vi "MesswertePlotten.vi"(0 "Intensity 0-100":dbl(knob) min=0.0 max=100.0 step=1.0 scale=0.0..100.0, 1 "VISA resource name":refnum<visa-resource-name>, 2 "file path (use dialog)":path, 3 "Upper colourlimit Temperatur":u32(colorbox), 4 "Lower colourlimit Temperatur":u32(colorbox), 5 "Upper colourlimit Humidity":u32(colorbox), 6 "Lower colourlimit Humidity":u32(colorbox)) -> ()   [LabVIEW 2021]
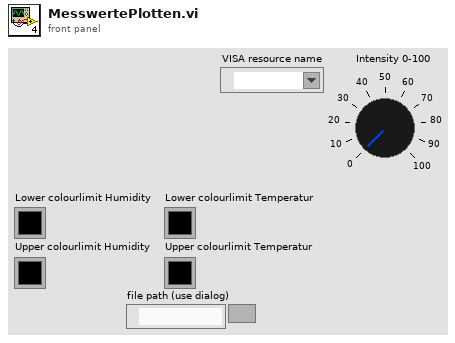
[diagram p1: front panel]
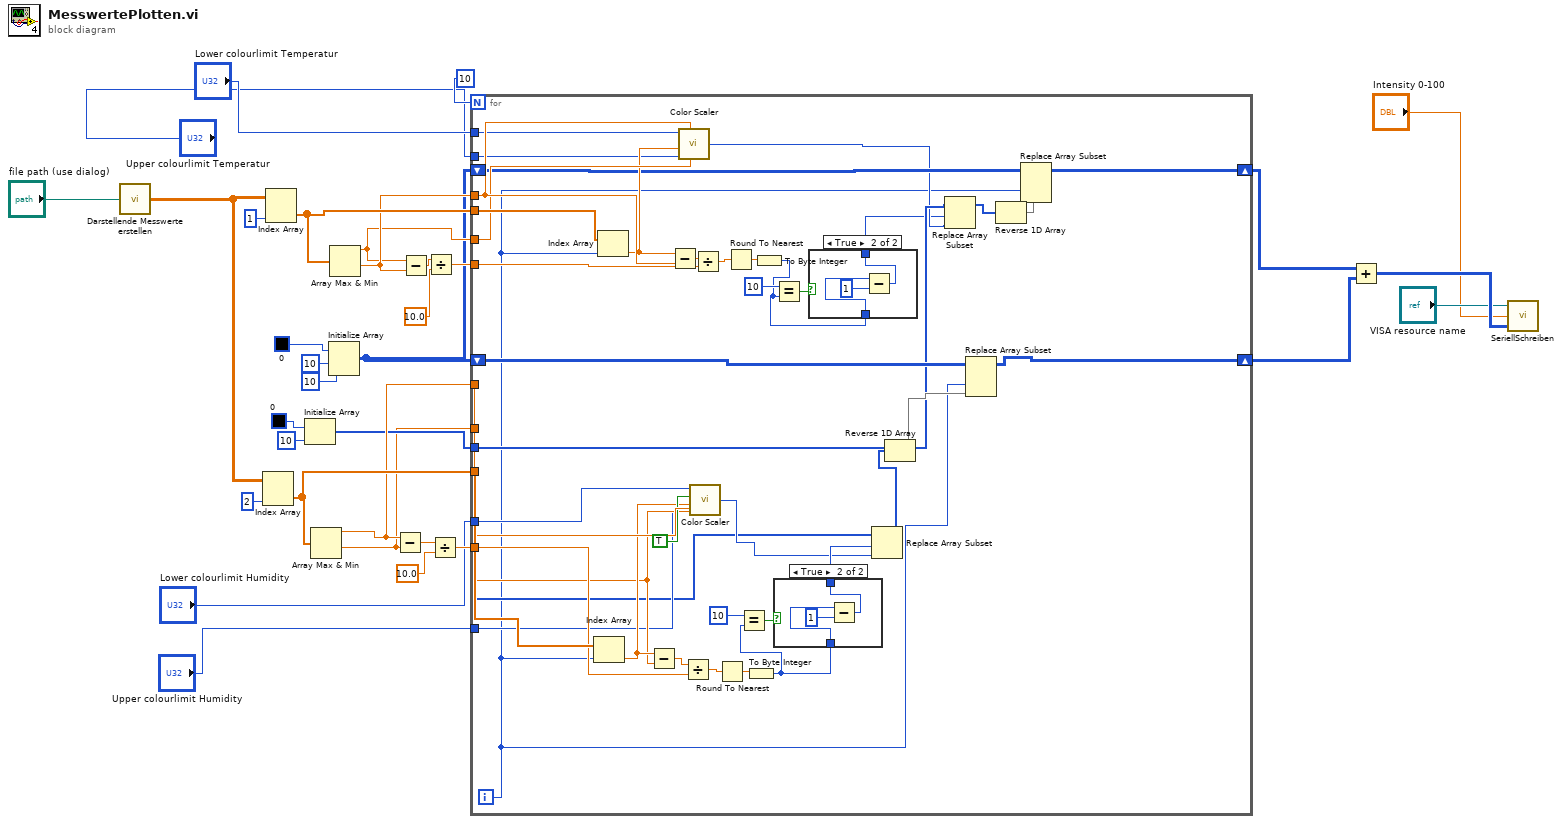
[diagram p0: block diagram]
diagram:
  n1 = call "Darstellende Messwerte erstellen.vi"("file path (use dialog)"="file path (use dialog)") -> ("output array"=w8:dbl[][])
  n2 = Index Array(array=w8, index (col)=2 ("disabled index (col)")) -> (element=w30:dbl[])  [unwired: 1 in]
  n3 = Index Array(array=w8, index (col)=1 ("disabled index (col)")) -> (element=w19:dbl[])  [unwired: 1 in]
  n4 = Initialize Array(u32 0 ("Output Color"), 10 ("dimension size")) -> (w17:u32[])
  n5 = Array Max & Min(array=w30) -> (max value=w23:dbl, min value=w15:dbl)  [unwired: 2 out]
  n6 = Initialize Array(u32 0 ("Output Color"), 10 ("dimension size"), 10 ("dimension size")) -> (w6:u32[][])
  n7 = Array Max & Min(array=w19) -> (max value=w13:dbl, min value=w14:dbl)  [unwired: 2 out]
  n8 = Subtract(x=w23, y=w15) -> (x-y=w29:dbl)
  n9 = Subtract(x=w13, y=w14) -> (x-y=w26:dbl)
  n10 = Divide(x=w26, y=10.0) -> (x/y=w24:dbl)
  n11 = Divide(x=w29, y=10.0) -> (x/y=w27:dbl)
  n12 = for {
    N: 10 -> [_]
    tunnel: w30 -> [w74]
    shift-right: [w45] -> w4
    shift-left: w6 -> [w44]
    tunnel: w27 -> [w73]
    tunnel: w24 -> [w58]
    tunnel: w15 -> [w61]
    tunnel: w23 -> [w72]
    tunnel: w19 -> [w60]
    tunnel: w13 -> [w54]
    tunnel: w14 -> [w55]
    tunnel: w17 -> [w41]
    tunnel: "Lower colourlimit Humidity" -> [w51]
    tunnel: "Upper colourlimit Humidity" -> [w50]
    tunnel: "Lower colourlimit Temperatur" -> [w49]
    tunnel: "Upper colourlimit Temperatur" -> [w48]
    shift-right: [w43] -> w5
    shift-left: w6 -> [w42]
    i -> [w34]
    n13 = Index Array(array=w74, index=w34) -> (element=w62:dbl)
    n14 = Index Array(array=w60, index=w34) -> (element=w53:dbl)
    n15 = Subtract(x=w62, y=w61) -> (x-y=w63:dbl)
    n16 = Subtract(x=w53, y=w55) -> (x-y=w59:dbl)
    n17 = call "Color Scaler.vi"("Upper numberlimit (default 30)"=w54, "Lower numberlimit (default 18)"=w55, "Upper colourlimit"=w48, "Input"=w53, "Lower colourlimit"=w49) -> ("Output Color"=w40:u32)  [unwired: 1 in]
    n18 = Divide(x=w63, y=w73) -> (x/y=w69:dbl)
    n19 = call "Color Scaler.vi"("Upper numberlimit (default 30)"=w72, "Lower numberlimit (default 18)"=w61, "Upper colourlimit"=w50, "Input"=w62, "Boolean (False =Temp;True=hum)"=TRUE, "Lower colourlimit"=w51) -> ("Output Color"=w47:u32)
    n20 = Divide(x=w59, y=w58) -> (x/y=w57:dbl)
    n21 = Round To Nearest(number=w69) -> (nearest integer value=w68:dbl)
    n22 = Round To Nearest(number=w57) -> (nearest integer value=w56:dbl)
    n23 = To Byte Integer(number=w68) -> (8bit integer=w66:i8)
    n24 = Equal?(x=i8 10, y=w66) -> (x = y?=w64:bool)
    n25 = To Byte Integer(number=w56) -> (8bit integer=w36:i8)
    n26 = Equal?(x=i8 10, y=w36) -> (x = y?=w37:bool)
    n27 = case shown="True" w64 {
      tunnel: w66 -> [w79 w82]
      tunnel: [w79 w80] -> w67
      frame False {
      }
      frame True {
        n28 = Subtract(x=w82, y=i8 1) -> (x-y=w80:i8)
      }
    }
    n29 = case shown="True" w37 {
      tunnel: w36 -> [w75 w78]
      tunnel: [w75 w76] -> w35
      frame False {
      }
      frame True {
        n30 = Subtract(x=w78, y=i8 1) -> (x-y=w76:i8)
      }
    }
    n31 = Replace Array Subset(array=w41, new element=w47, index=w67) -> (w70:u32[])
    n32 = Reverse 1D Array(array=w70) -> (reversed array=w46:u32[])
    n33 = Replace Array Subset(array=w41, new element=w40, index=w35) -> (w39:u32[])
    n34 = Replace Array Subset(array=w44, new element=w46, index (col)=w34) -> (w45:u32[][])  [unwired: 1 in]
    n35 = Reverse 1D Array(array=w39) -> (reversed array=w52:u32[])
    n36 = Replace Array Subset(array=w42, new element=w52, index (col)=w34) -> (w43:u32[][])  [unwired: 1 in]
  }
  n37 = Add(x=w5, y=w4) -> (x+y=w3:u32[][])
  n38 = call "SeriellSchreiben.vi"("Array 100*100 rgb"=w3, "Intensity 0-100"="Intensity 0-100", "VISA resource name"="VISA resource name") -> ()  [unwired: 1 out]
